vi "FTW-Connector-SendPoisonPill.vi"(0 "FTW Actor Connector":refnum<class "FTW-ActorConnector.lvclass">, 11 "error in":errorcluster) -> (4 "FTW Actor Connector out":refnum<class "FTW-ActorConnector.lvclass">, 15 "error out":errorcluster)   [LabVIEW 2012, in "FTW-Actor.lvlib" / "FTW-ActorConnector.lvclass"]
uses:
  FTW-ActorConnector.lvclass
panel:
  # "Inputs"
  # "Outputs"
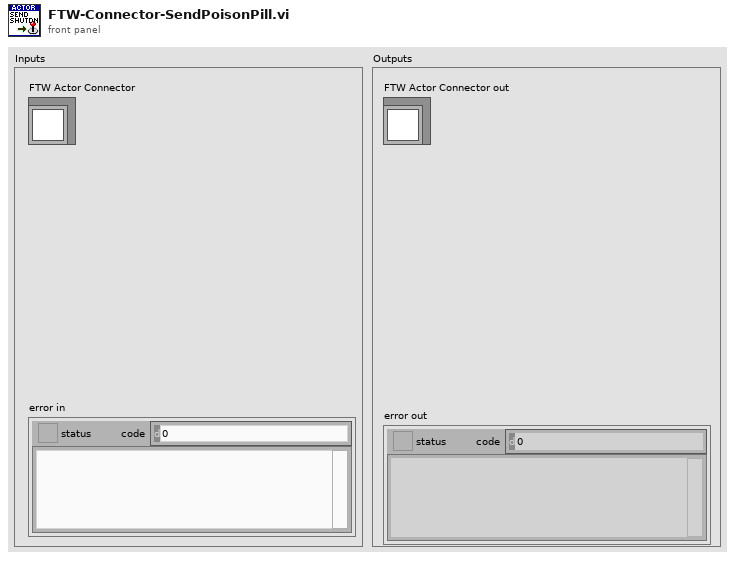
[diagram p1: front panel]
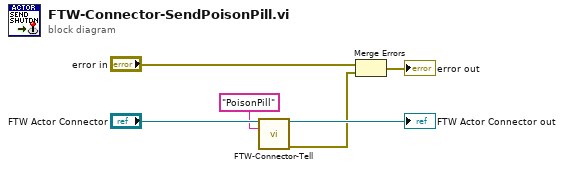
[diagram p0: block diagram]
diagram:
  n1 = call "FTW-Connector-Tell.vi"("FTW Actor Reference"="FTW Actor Connector", "Message Header"="PoisonPill" ("Message")) -> ("FTW Actor Reference out"=→"FTW Actor Connector out":refnum<class "FTW-ActorConnector.lvclass">, "error out"=w1:errorcluster)  [unwired: 11 in, 1 out]
  n2 = Merge Errors("error in", w1) -> (→"error out":errorcluster)
